vi "mpps_keithley-2450_python.vi"(0 "start voltage (V)":string, 1 "file name":string, 2 "folder path":string, 5 "nplc":string, 7 "settling delay (s)":string, 9 "total tracking time (s)":string, 11 "error in (no error)":errorcluster, 12 "illumination intensity (suns equiv.)":string, 13 "area (cm^2)":string) -> (15 "error out":errorcluster)   [LabVIEW 2016]
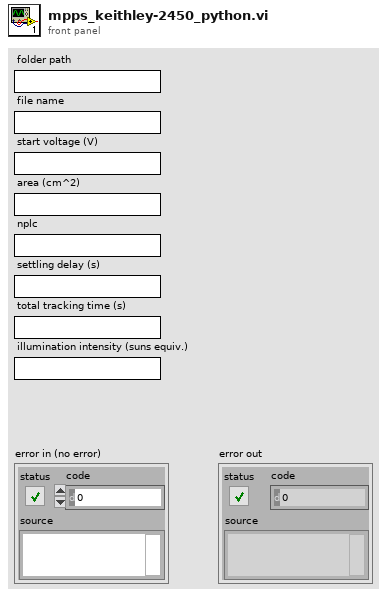
[diagram p1: front panel]
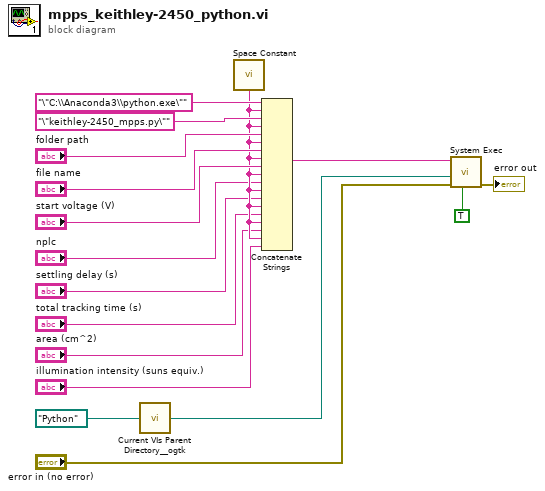
[diagram p0: block diagram]
diagram:
  n1 = call <userlib>:"Current VIs Parent Directory__ogtk.vi"("Relative path (.)"=path "Python") -> ("Parent Directory (+ Relative)"=w1:path)  [unwired: 4 in]
  n2 = call <vilib>:"Space Constant.vi"() -> ("String"=w8:string)
  n3 = Concatenate Strings("\"C:\\Anaconda3\\python.exe\"" ("standard input"), w8, "\"keithley-2450_mpps.py\"" ("standard input"), w8, "folder path", w8, "file name", w8, "start voltage (V)", w8, "nplc", w8, "settling delay (s)", w8, "total tracking time (s)", w8, "area (cm^2)", w8, "illumination intensity (suns equiv.)") -> (w15:string)
  n4 = call <vilib>:"System Exec.vi"("run minimized? (F)"=TRUE, "error in (no error)"="error in (no error)", "working directory"=w1, "command line"=w15) -> ("error out"=→"error out":errorcluster)  [unwired: 4 in, 3 out]
